vi "Delete Operation and Display Update.vi"(8 "error in (no error)":errorcluster, 10 "Previous Index IN":i32, 11 "UI control refnums":T1) -> (0 "error out":errorcluster, 3 "New Index OUT":i32, 4 "Macro Error OUT":bool)   [LabVIEW 2012]
doc: "SciScan 1.2 160622"
uses:
  Custom Controls and Typedefs/Macro_MD_UI Control Refnums.ctl
  Custom Controls and Typedefs/Delete Button.ctl
  Custom Controls and Typedefs/Edit Button.ctl
  Custom Controls and Typedefs/Timing Estimate Cluster.ctl
  CommonResource VIs/Timing/Timing Indicator.ctl
  Custom Controls and Typedefs/Load from PSM Button.ctl
  CommonResource VIs/FormatTree&TableStyle_Commands.ctl
  Macro Loop Manager Module/SubVIs/Macro Execution and Timing_Commands.ctl
  SubVIs/FGV_MacroCore_Commands.ctl
panel:
  # "(hh:mm:ss)"
  # "(hh:mm:ss)"
  # "(hh:mm:ss)"
  # "(hh:mm:ss)"
  # "(hh:mm:ss)"
  # "(hh:mm:ss)"
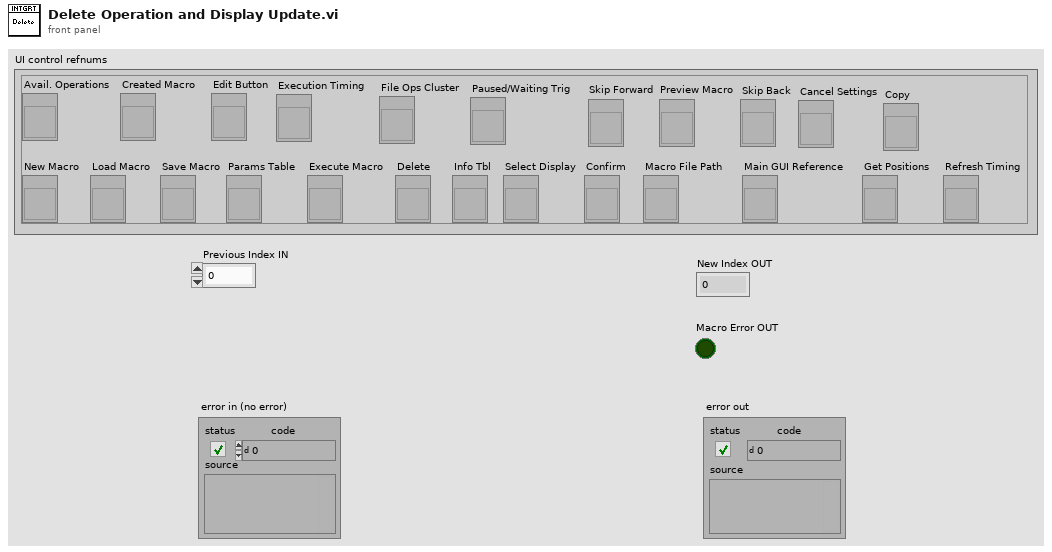
[diagram p1: front panel]
types:
  T1 = typedef "Macro_MD_UI Control Refnums.ctl" = cluster{"Avail. Operations":refnum<vi>, "Created Macro":refnum<vi>, "Load Macro":refnum<vi>, "Save Macro":refnum<vi>, "Params Table":refnum<vi>, "Delete":refnum<vi>, "Edit Button":refnum<vi>, "Execute Macro":refnum<vi>, "Info Tbl":refnum<vi>, "Execution Timing":refnum<vi>, "Select Display":refnum<vi>, "File Ops Cluster":refnum<vi>, "Paused/Waiting Trig":refnum<vi>, "Confirm":refnum<vi>, "New Macro":refnum<vi>, "Preview Macro":refnum<vi>, "Skip Forward":refnum<vi>, "Skip Back":refnum<vi>, "Macro File Path":refnum<vi>, "Main GUI Reference":refnum<vi>, "Cancel Settings":refnum<vi>, "Get Positions":refnum<vi>, "Copy":refnum<vi>, "Refresh Timing":refnum<vi>}
  T2 = typedef "FormatTree&TableStyle_Commands.ctl" = enum16{"Colour Row", "Uncolour Row", "Bold Row", "Unbold Row", "Clear", "UpdateVisibleRows"}
  T3 = typedef "Macro Execution and Timing_Commands.ctl" = enum16{"Initialize (Update FGV & Rst Idx)", "Run", "EstimateTime", "Preview", "Update Macro array (Idx Unchanged)", "Update Index", "Clear Timing Info"}
  T4 = typedef "FGV_MacroCore_Commands.ctl" = enum16{"Initialize", "Get Array", "Load macro from file", "Insert Item", "Insert at End", "Edit Parameter String", "Delete instruction", "Move Items", "Save", "SaveAs", "UpdateInfoTable", "Edit Settings File", "New Macro", "Read Temp File", "Delete Multiple"}
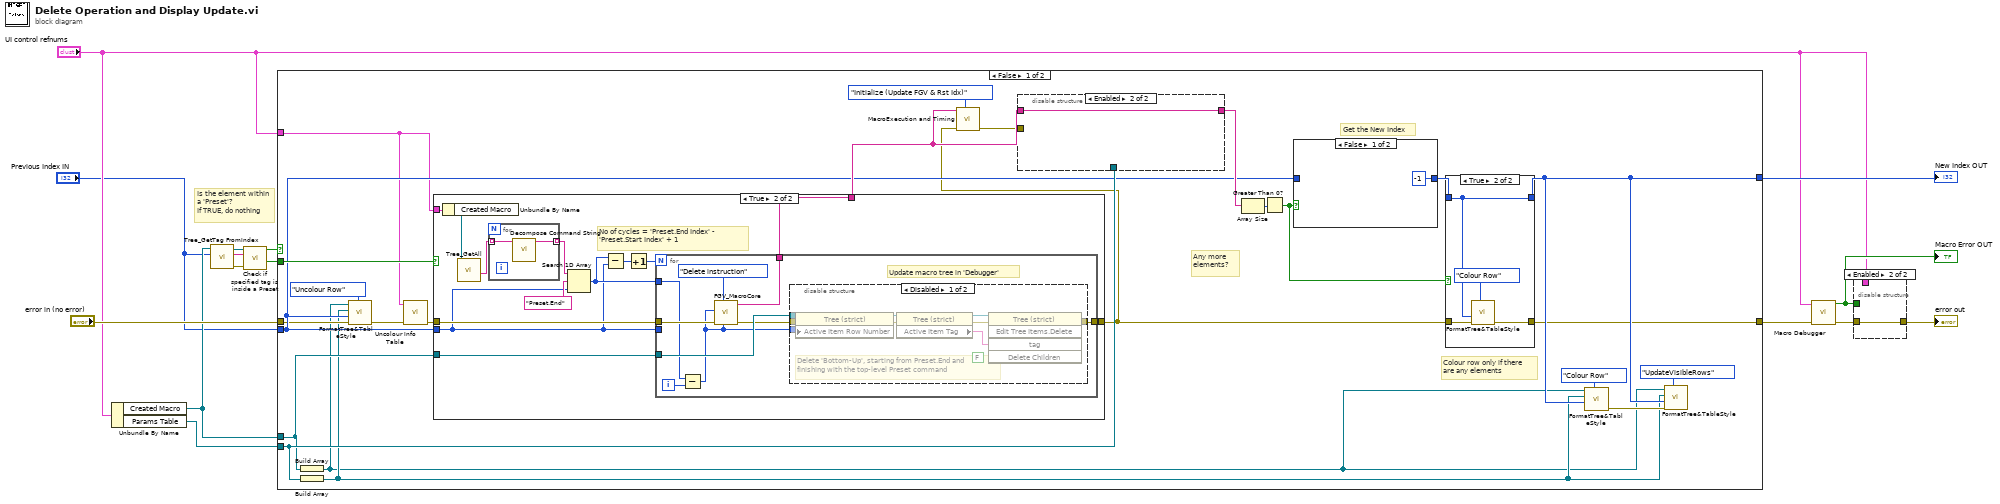
[diagram p0: block diagram]
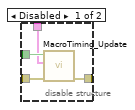
[diagram p2: hidden frame]
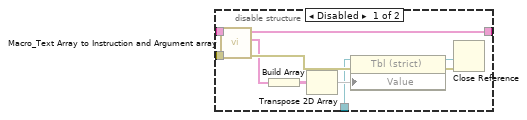
[diagram p3: hidden frame]
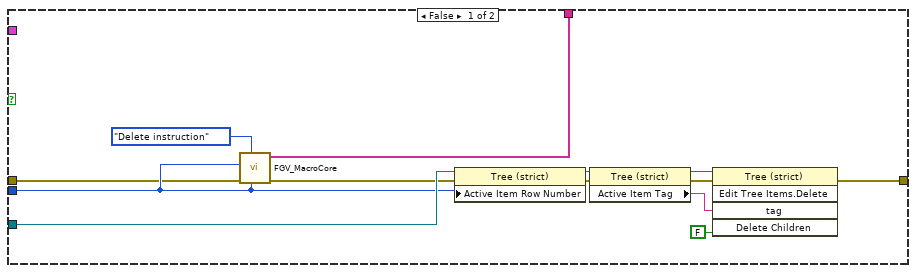
[diagram p4: hidden frame]
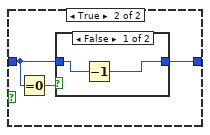
[diagram p6: hidden frame]
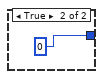
[diagram p7: hidden frame]
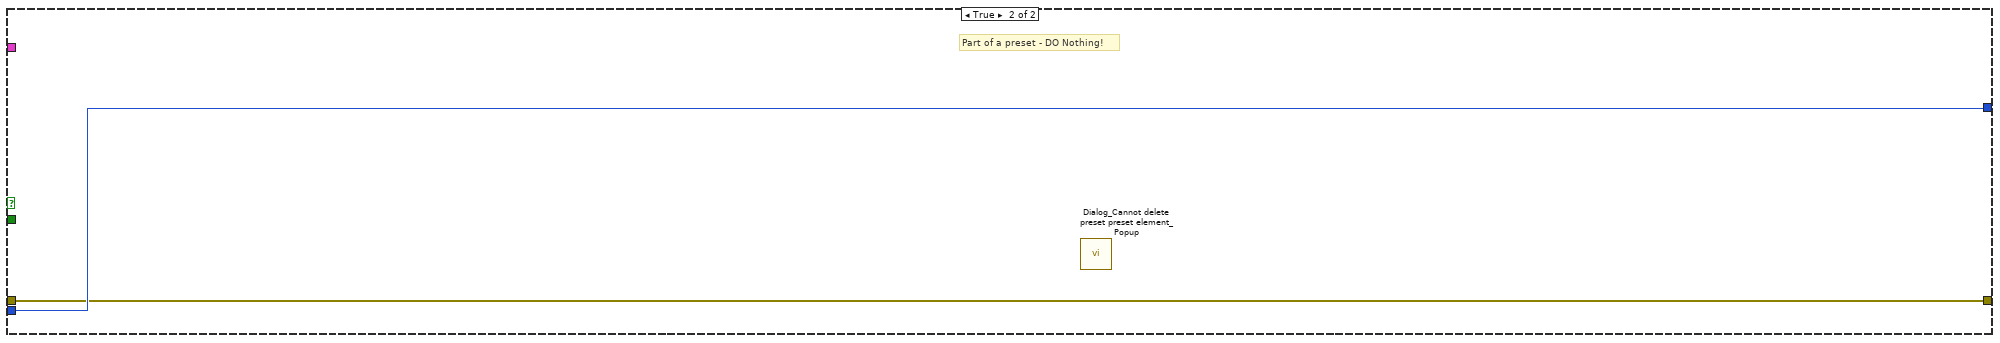
[diagram p9: hidden frame]
diagram:
  # "Is the element within a 'Preset'?\nIf TRUE, do nothing"
  n1 = Unbundle By Name("UI control refnums") -> ("Created Macro"=w7:refnum<vi>, "Params Table"=w15:refnum<vi>)
  n2 = call "Tree_GetTag FromIndex.vi"("Index IN"="Previous Index IN", "Tree Refnum IN"=w7) -> ("Error Out"=w3:errorcluster, "Tag OUT"=w5:string, "Tree Refnum OUT"=w4:refnum<vi>)  [unwired: 7 in]
  n3 = call "Check if specified tag is inside a Preset.vi"("error in (no error)"=w3, "Tag to check"=w5, "Tree Refnum"=w4) -> ("Specified Tag is a Preset command?"=w1:bool, "Specified tag is part of a Preset?"=w2:bool)  [unwired: 5 in, 2 out]
  n4 = case shown="False" w2 {
    tunnel: w15 -> [w32 _]
    tunnel: "error in (no error)" -> [w22 w112]
    tunnel: [w31 w113] -> w13
    tunnel: [w28 w112] -> w12
    tunnel: "UI control refnums" -> [w16 _]
    tunnel: w7 -> [w26 _]
    tunnel: "Previous Index IN" -> [w23 w113]
    tunnel: w1 -> [w25 _]
    frame False {
      # "Get the New Index"
      # "Any more elements?"
      # "Colour row only if there\nare any elements"
      n5 = Build Array(w26) -> (w20:refnum<vi>[])
      n6 = Build Array(w32) -> (w21:refnum<vi>[])
      n7 = call "FormatTree&TableStyle.vi"("Format Command"=FormatTree&TableStyle_Commands."Uncolour Row", "Error In"=w22, "Row Index"=w23, "Array of Table references"=w21, "Array of Tree references"=w20) -> ("Error Out"=w19:errorcluster)  [unwired: 6 in]
      n8 = call "Uncolour Info Table.vi"("Error In"=w19, "UI control refnums"=w16) -> ("Error Out"=w18:errorcluster)  [unwired: 9 in]
      n9 = case shown="True" w25 {
        tunnel: [w56 w76] -> w17
        tunnel: [w55 w75] -> w29
        tunnel: w26 -> [w54 w74]
        tunnel: w23 -> [w53 w68]
        tunnel: w18 -> [w52 w73]
        tunnel: w16 -> [_ w72]
        frame False {
          n10 = call "FGV_MacroCore.vi"("Final Index"=w53, "MacroFGV_Commands"=FGV_MacroCore_Commands."Delete instruction", "Error In"=w52, "Start Index"=w53) -> ("Error Out"=w51:errorcluster, "Macro String Array"=w55:string[])  [unwired: 3 in, 3 out]
          n11 = property class="Tree (strict)"(reference=w54, error in=w51, "Active Item Row Number"=w53) -> (reference out=w62:refnum<vi>, error out=w61:errorcluster)
          n12 = property class="Tree (strict)"(reference=w62, error in=w61) -> (reference out=w57:refnum<vi>, error out=w59:errorcluster, "Active Item Tag"=w60:string)
          n13 = invoke class="Tree (strict)" method="Edit Tree Items.Delete"(reference=w57, error in=w59, "tag"=w60, "Delete Children"=FALSE ("Delete Children?")) -> (error out=w56:errorcluster)  [unwired: 1 in, 4 out]
        }
        frame True {
          # "No of cycles = 'Preset.End Index' - 'Preset.Start Index' + 1"
          n14 = Unbundle By Name(w72) -> ("Created Macro"=w71:refnum<vi>)
          n15 = call "Tree_GetAll.vi"("Tree Refnum IN"=w71) -> ("Text"=w65:string[])  [unwired: 7 in, 3 out]
          n16 = for {
            tunnel: w65 -> [w78] mode=indexing
            tunnel: [w77] -> w64 mode=indexing
            n17 = call "Decompose Command String.vi"("Command IN"=w78) -> ("Action"=w77:string)  [unwired: 7 in, 3 out]
          }
          n18 = Search 1D Array(1D array=w64, element="Preset.End", start index (0)=w68) -> (index of element=w69:i32)
          n19 = Subtract(x=w69, y=w68) -> (x-y=w67:i32)
          n20 = Increment(x=w67) -> (x+1=w66:i32)
          n21 = for {
            N: w66 -> [_]
            tunnel: [w86] -> w76
            tunnel: [w85] -> w75
            tunnel: w74 -> [w84]
            tunnel: w73 -> [w83]
            tunnel: w68 -> [_]
            tunnel: w69 -> [w80]
            i -> [w81]
            # "Update macro tree in 'Debugger'"
            n22 = Subtract(x=w80, y=w81) -> (x-y=w79:i32)
            n23 = call "FGV_MacroCore.vi"("Final Index"=w79, "MacroFGV_Commands"=FGV_MacroCore_Commands."Delete instruction", "Error In"=w83, "Start Index"=w79) -> ("Error Out"=w82:errorcluster, "Macro String Array"=w85:string[])  [unwired: 3 in, 3 out]
            n24 = disable-structure shown="Disabled" {
              disable-tunnel: [w91 w98] -> w86
              disable-tunnel: w84 -> [w90 _]
              disable-tunnel: w82 -> [w89 w98]
              disable-tunnel: w79 -> [w88 _]
              frame Disabled {
                # "Delete 'Bottom-Up', starting from Preset.End and finishing with the top-level Preset command"
                n25 = property class="Tree (strict)"(reference=w90, error in=w89, "Active Item Row Number"=w88) -> (reference out=w97:refnum<vi>, error out=w96:errorcluster)
                n26 = property class="Tree (strict)"(reference=w97, error in=w96) -> (reference out=w92:refnum<vi>, error out=w94:errorcluster, "Active Item Tag"=w95:string)
                n27 = invoke class="Tree (strict)" method="Edit Tree Items.Delete"(reference=w92, error in=w94, "tag"=w95, "Delete Children"=FALSE ("Delete Children?")) -> (error out=w91:errorcluster)  [unwired: 1 in, 4 out]
              }
              frame Enabled {
              }
            }
          }
        }
      }
      n28 = call "MacroExecution and Timing.vi"("MacroExecution and Timing Command"=Macro_Execution_and_Timing_Commands."Initialize (Update FGV & Rst Idx)", "Error In"=w17, "Macro IN"=w29) -> ("Error Out"=w27:errorcluster)  [unwired: 3 in, 5 out]
      n29 = disable-structure shown="Enabled" {
        disable-tunnel: [w43 w50] -> w37
        disable-tunnel: w32 -> [w42 _]
        disable-tunnel: w29 -> [w41 w50]
        disable-tunnel: w27 -> [w40 _]
        frame Disabled {
          n30 = call "Macro_Text Array to Instruction and Argument array.vi"("Error In"=w40, "Macro Array IN"=w41) -> ("Error Out"=w45:errorcluster, "Argument List (Txt)"=w44:string[], "Action List (Txt)"=w43:string[])  [unwired: 7 in]
          n31 = Build Array(w44) -> (w49:string[][])
          n32 = Transpose 2D Array(2D array=w49) -> (transposed array=w48:string[][])
          n33 = property class="Tbl (strict)"(reference=w42, error in=w45, "Value"=w48) -> (reference out=w46:refnum<vi>, error out=w47:errorcluster)
          n34 = Close Reference(reference=w46, error in (no error)=w47) -> ()  [unwired: 1 out]
        }
        frame Enabled {
        }
      }
      n35 = Array Size(array=w37) -> (size(s)=w33:i32)
      n36 = Greater Than 0?(x=w33) -> (x > 0?=w38:bool)
      n37 = case shown="False" w38 {
        tunnel: w23 -> [_ w101]
        tunnel: [-1 ("Index") w100] -> w39
        frame False {
        }
        frame True {
          n38 = Equal To 0?(x=w101) -> (x = 0?=w102:bool)
          n39 = case shown="False" w102 {
            tunnel: w101 -> [w104 _]
            tunnel: [w103 0 ("Index")] -> w100
            frame False {
              n40 = Decrement(x=w104) -> (x-1=w103:i32)
            }
            frame True {
            }
          }
        }
      }
      n41 = case shown="True" w38 {
        tunnel: w17 -> [w107 w110]
        tunnel: w39 -> [w106 w108]
        tunnel: [w107 w109] -> w28
        tunnel: [w106 w108] -> w31
        frame False {
          # "Index = 0 if only\n1 element. If no\n elements,\nindex = -1"
        }
        frame True {
          n42 = call "FormatTree&TableStyle.vi"("Format Command"=FormatTree&TableStyle_Commands."Colour Row", "Error In"=w110, "Row Index"=w108) -> ("Error Out"=w109:errorcluster)  [unwired: 8 in]
        }
      }
      n43 = call "FormatTree&TableStyle.vi"("Format Command"=FormatTree&TableStyle_Commands."Colour Row", "Row Index"=w31, "Array of Table references"=w21, "Array of Tree references"=w20) -> ("Error Out"=w35:errorcluster)  [unwired: 7 in]
      n44 = call "FormatTree&TableStyle.vi"("Format Command"=FormatTree&TableStyle_Commands."UpdateVisibleRows", "Error In"=w35, "Row Index"=w31, "Array of Table references"=w21, "Array of Tree references"=w20) -> ()  [unwired: 6 in, 1 out]
    }
    frame True {
      # "Part of a preset - DO Nothing!"
      n45 = call "Dialog_Cannot delete preset preset element_Popup.vi"() -> ()  [unwired: 11 in, 1 out]
    }
  }
  "New Index OUT" <- w13
  n46 = call "Macro Debugger.vi"("Error In"=w12, "UI control refnums"="UI control refnums") -> ("Error Out"=w11:errorcluster, "Any Error?"=w10:bool)  [unwired: 8 in]
  "Macro Error OUT" <- w10
  n47 = disable-structure shown="Enabled" {
    disable-tunnel: w11 -> [w117 w118]
    disable-tunnel: w10 -> [w116 _]
    disable-tunnel: "UI control refnums" -> [w115 _]
    disable-tunnel: [w114 w118] -> w8
    frame Disabled {
      n48 = call "MacroTiming_Update.vi"("error in (no error)"=w117, "UI control refnums"=w115, "Macro Error IN?"=w116) -> ("error out"=w114:errorcluster)  [unwired: 8 in]
    }
    frame Enabled {
    }
  }
  "error out" <- w8
